vi "Publish Data.vi"() -> (0 "error out":errorcluster, 4 "log":string)   [LabVIEW 2024]
uses:
  <vilib>/Plug-In SDKs/Clients/Data Store V1/Data Store Client.lvlibp/API/Data Store V1/Test Result.ctl
  <vilib>/Plug-In SDKs/Clients/Metadata/Outcome.ctl
  <vilib>/Plug-In SDKs/Clients/Metadata/Extension.ctl
  Test Result Info.ctl
  <vilib>/Plug-In SDKs/Clients/Metadata/Step.ctl
  <vilib>/numeric/Random Number (Range) DBL.vi
  <vilib>/Plug-In SDKs/Clients/Data Store V1/Data Store Client.lvlibp/API/Data Store V1/Publish Measurement (DBL).vi
  <vilib>/Plug-In SDKs/Clients/Data Store V1/Data Store Client.lvlibp/API/Data Store V1/Publish Condition (Double).vi
  <vilib>/Plug-In SDKs/Clients/Data Store V1/Data Store Client.lvlibp
  <vilib>/Plug-In SDKs/Clients/Metadata/NI Metadata Types.lvlib
panel:
  # "Publish Data\n\nCreates and publishes data and metadata items that can be queried using the other VIs in this example."
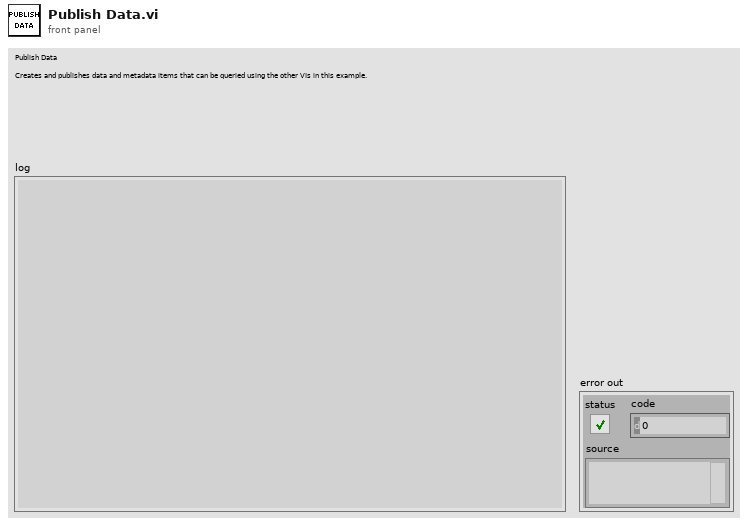
[diagram p1: front panel]
types:
  T1 = typedef "Data Store Client.lvlibp/Test Result.ctl" = cluster{"test result name":string, "start date time":timestamp, "end date time":timestamp, "outcome":T2, "test result id":string, "uut instance id":string, "operator id":string, "test station id":string, "test description id":string, "software item ids":string[], "hardware item ids":string[], "test adapter ids":string[], "link":string, "extensions":T3[], "schema id":string}
  T2 = typedef "NI Metadata Types.lvlib/Outcome.ctl" = enum32{"Unspecified", "Passed", "Failed", "Indeterminate"}
  T3 = typedef "NI Metadata Types.lvlib/Extension.ctl" = cluster{"name":string, "value":string}
  T4 = typedef "Test Result Info.ctl" = cluster{"Name":string, "Measurements":cluster{"Name":string, "Min_Value":dbl, "Max_Value":dbl, "Units":string}[], "Conditions":cluster{"Name":string, "Min_Value":dbl, "Max_Value":dbl, "Units":string}[]}[]
  T5 = typedef "NI Metadata Types.lvlib/Step.ctl" = cluster{"step name":string, "step type":string, "start date time":timestamp, "end date time":timestamp, "notes":string, "step id":string, "parent step id":string, "test result id":string, "test id":string, "link":string, "extensions":T3[], "schema id":string}
  T6 = cluster{"Name":string, "Min_Value":dbl, "Max_Value":dbl, "Units":string}[]
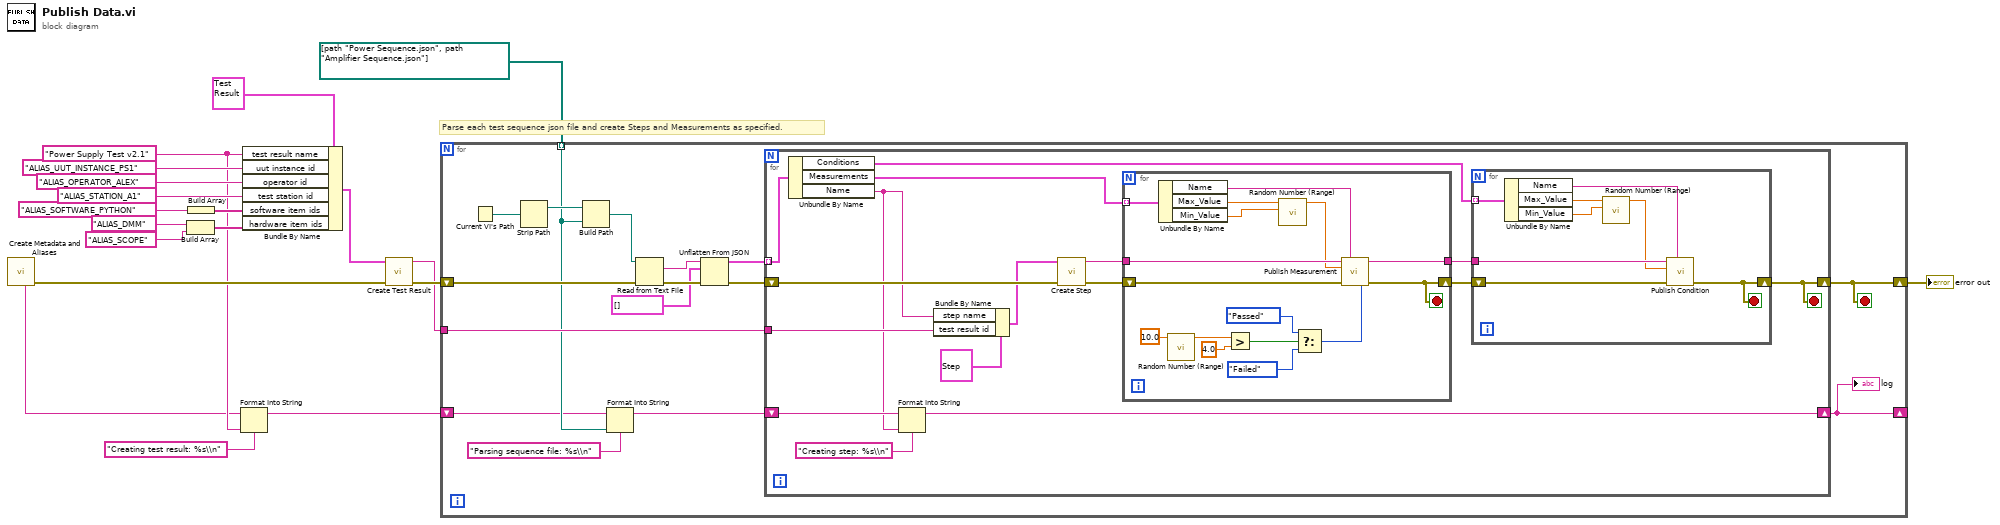
[diagram p0: block diagram]
diagram:
  w3 = "Power Supply Test v2.1" ("test result name")
  # "Parse each test sequence json file and create Steps and Measurements as specified."
  n1 = call "Create Metadata and Aliases.vi"() -> ("error out"=w9:errorcluster, "log"=w2:string)  [unwired: 10 in]
  n2 = Build Array("ALIAS_DMM" ("test station id"), "ALIAS_SCOPE" ("element")) -> (w12:string[])
  n3 = Build Array("ALIAS_SOFTWARE_PYTHON" ("test station id")) -> (w14:string[])
  n4 = Format Into String(format string="Creating test result: %s\\n", initial string=w2, w3) -> (resulting string=w1:string)  [unwired: 1 in, 1 out]
  n5 = Bundle By Name(cluster=T1 {"test result name"="", "start date time"=timestamp(0 s since 1904-01-01), "end date time"=timestamp(0 s since 1904-01-01), "outcome"=enum."Unspecified", "test result id"="", "uut instance id"="", "operator id"="", "test station id"="", "test description id"="", "software item ids"=[], "hardware item ids"=[], "test adapter ids"=[], "link"="", "extensions"=[], "schema id"=""} ("test result"), "test result name"=w3, "uut instance id"="ALIAS_UUT_INSTANCE_PS1", "operator id"="ALIAS_OPERATOR_ALEX", "test station id"="ALIAS_STATION_A1", "software item ids"=w14, "hardware item ids"=w12) -> (w10:T1)
  n6 = call <vilib>:"Create Test Result.vi"("error in"=w9, "test result"=w10) -> ("error out"=w8:errorcluster, "test result id"=w6:string)  [unwired: 8 in]
  n7 = for {
    tunnel: path[] [path "Power Sequence.json", path "Amplifier Sequence.json"] -> [w24] mode=indexing
    tunnel: w6 -> [w27]
    shift-right: [w21] -> w5
    shift-left: w8 -> [w35]
    shift-right: [w20] -> _
    shift-left: w1 -> [w23]
    stop <- w21 stop-if-true
    n8 = Current VI's Path() -> (path=w34:path)
    n9 = Strip Path(path=w34) -> (stripped path=w33:path)  [unwired: 1 out]
    n10 = Build Path(base path=w33, name or relative path=w24) -> (appended path=w32:path)
    n11 = Format Into String(format string="Parsing sequence file: %s\\n", initial string=w23, w24) -> (resulting string=w22:string)  [unwired: 1 in, 1 out]
    n12 = Read from Text File(file (use dialog)=w32, error in=w35) -> (text=w30:string, error out=w31:errorcluster)  [unwired: 2 in, 2 out]
    n13 = Unflatten From JSON(JSON string=w30, type and defaults=T4 [] ("Steps"), error in (no error)=w31) -> (value=w28:T4, error out=w29:errorcluster)  [unwired: 4 in]
    n14 = for {
      shift-right: [w36] -> w21
      shift-left: w29 -> [w50]
      tunnel: w28 -> [w51] mode=indexing
      tunnel: w27 -> [w48]
      shift-right: [w37] -> w20
      shift-left: w22 -> [w40]
      stop <- w36 stop-if-true
      n15 = Unbundle By Name(w51) -> ("Conditions"=w41:T6, "Measurements"=w46:T6, "Name"=w38:string)
      n16 = Format Into String(format string="Creating step: %s\\n", initial string=w40, w38) -> (resulting string=w37:string)  [unwired: 1 in, 1 out]
      n17 = Bundle By Name(cluster=T5 {"step name"="", "step type"="", "start date time"=timestamp(0 s since 1904-01-01), "end date time"=timestamp(0 s since 1904-01-01), "notes"="", "step id"="", "parent step id"="", "test result id"="", "test id"="", "link"="", "extensions"=[], "schema id"=""} ("step"), "step name"=w38, "test result id"=w48) -> (w47:T5)
      n18 = call <vilib>:"Create Step.vi"("error in"=w50, "step"=w47) -> ("error out"=w43:errorcluster, "step id"=w45:string)  [unwired: 8 in]
      n19 = for {
        tunnel: w46 -> [w75] mode=indexing
        tunnel: w45 -> [w73]
        tunnel: [w69] -> w44
        shift-right: [w60] -> w42
        shift-left: w43 -> [w68]
        stop <- w60 stop-if-true
        n20 = Unbundle By Name(w75) -> ("Name"=w74:string, "Max_Value"=w72:dbl, "Min_Value"=w71:dbl)
        n21 = call-poly <vilib>:"Random Number (Range).vi"("upper bound (100)"=10.0) -> ("number"=w66:dbl)  [unwired: 10 in]
        n22 = Greater?(x=w66, y=4.0) -> (0:w64:bool)
        n23 = call-poly <vilib>:"Random Number (Range).vi"("lower bound (0)"=w71, "upper bound (100)"=w72) -> ("number"=w70:dbl)  [unwired: 9 in]
        n24 = Select(t=Outcome."Passed" ("outcome"), s=w64, f=Outcome."Failed" ("outcome")) -> (s? t:f=w61:T2)
        n25 = call-poly <vilib>:"Publish Measurement.vi"("step id"=w73, "name"=w74, "outcome"=w61, "value"=w70, "error in"=w68) -> ("step id out"=w69:string, "error out"=w60:errorcluster)  [unwired: 8 in, 1 out]
      }
      n26 = for {
        tunnel: w41 -> [w59] mode=indexing
        tunnel: w44 -> [w57]
        shift-right: [w52] -> w36
        shift-left: w42 -> [w56]
        stop <- w52 stop-if-true
        n27 = Unbundle By Name(w59) -> ("Name"=w58:string, "Max_Value"=w55:dbl, "Min_Value"=w54:dbl)
        n28 = call-poly <vilib>:"Random Number (Range).vi"("lower bound (0)"=w54, "upper bound (100)"=w55) -> ("number"=w53:dbl)  [unwired: 9 in]
        n29 = call-poly <vilib>:"Publish Condition.vi"("name"=w58, "error in"=w56, "value"=w53, "step id"=w57) -> ("error out"=w52:errorcluster)  [unwired: 5 in, 2 out]
      }
    }
    "log" <- w20
  }
  "error out" <- w5
